vi "E727_Simple_Test.vi"(0 "System no.":i32=1 min=1 step=1, 2 "Interface":u16(ring) items=["RS232", "TCP/IP", "USB"], 3 "Timeout":u32=5000, 5 "error in":errorcluster, 6 "RS232 settings":cluster{"Portnumber":i32, "Baudrate":u16}={"Portnumber"=0, "Baudrate"=5} {"Baudrate" items=["9600", "14400", "19200", "38400", "57600", "115200"]; "Portnumber" items=["COM1", "COM2", "COM3", "COM4", "COM5", "COM6", "COM7", "COM8", "COM9", "COM10", "COM11", "COM12", "COM13", "COM14", "COM15", "COM16", "COM17", "COM18", "COM19", "COM20", "COM21", "COM22", "COM23", "COM24", "COM25", "COM26", "COM27", "COM28", "COM29", "COM30"]}, 7 "TCP/IP settings":T1={"Host address/name"="localhost", "Port"=50000, "Board"=0, "TCP/IP Search?"=TRUE}, 8 "USB settings":cluster{"S/N":string, "USB Search?":bool}={"S/N"="", "USB Search?"=TRUE}) -> (14 "Identification":string, 15 "Helpstring":string, 16 "Conn. Axes":string[](array[string]), 17 "Position":dbl[](array[numeric]) format="%.6f", 19 "error out":errorcluster)   [LabVIEW 2014]
doc: "This simple test VI is a stand-alone sample application. Use the \nHelp->Show Context Help menu sequence in the LabVIEW environment to display the Context Help window with the VI and control/indicator descriptions.\nSpecify \n- System no. (= 1 in a one-system configuration),\n- Interface (= RS232, TCP/IP or USB)\n- Timeout value (in milliseconds)\n- and interface settings first.\nThen start the VI. The VI will open a connection to the E-727 and query the controller for its identification string (*IDN?), help string (HLP?), the IDs (SAI?) and stage names (CST?) of the connected axes and their current position values (POS?). The diagram shows how to combine the driver and support VIs for these tasks."
panel:
  out "Stage names":string[](array[string])
  # "Simple E-727 communication test program"
  # "Select E-727 interface, timeout value and interface settings first, then start the VI. \nThe VI will open the chosen port, query for the connected axes (SAI?), the stage names (CST?), the position (POS?), Identification (*IDN?) and help string\n(HLP?). See VI and control/ indicator information for details."
  # "Only for\nInterface = \nTCP/IP:"
  # "Only for\nInterface = \nRS232:"
  # "Only for\nInterface = \nUSB:"
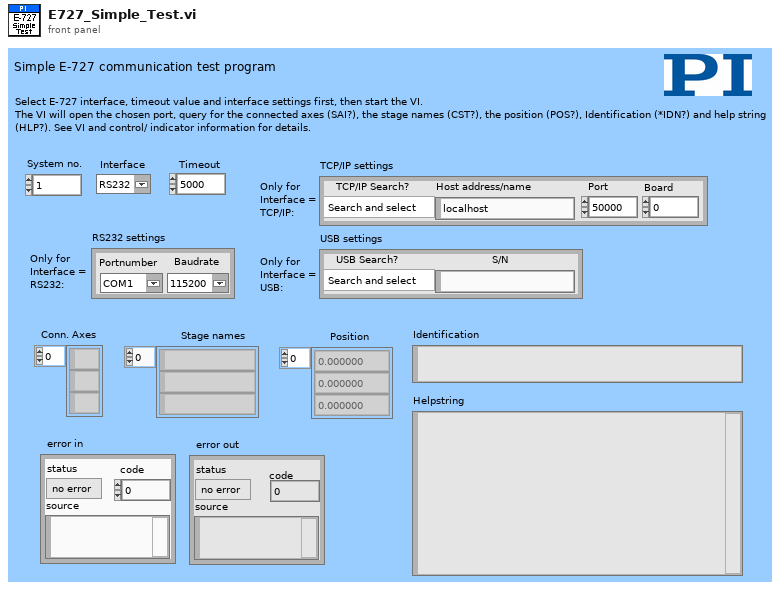
[diagram p1: front panel]
types:
  T1 = cluster{"Host address/name":string, "Port":i32, "Board":i32, "TCP/IP Search?":bool}
  T2 = cluster{"Host address/name":string, "Port":i32, "Board":i32}
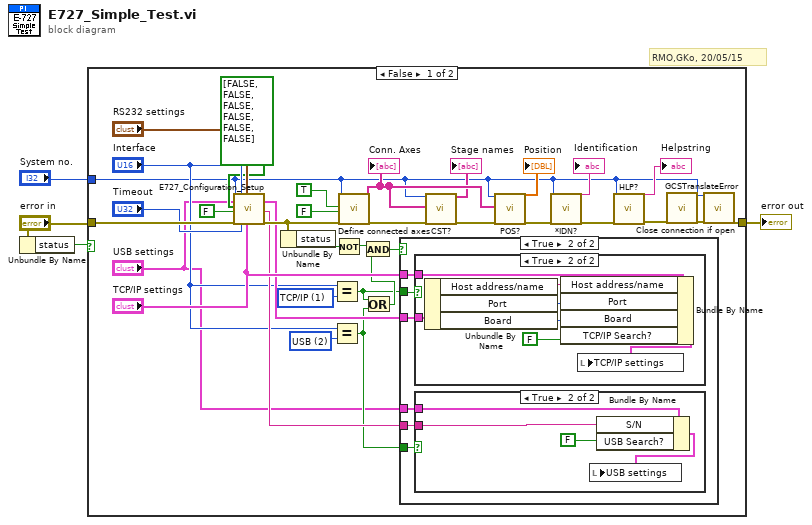
[diagram p0: block diagram]
diagram:
  # "RMO,GKo, 20/05/15"
  n1 = Unbundle By Name("error in") -> ("status"=w2:bool)
  n2 = case shown="False" w2 {
    tunnel: [w6 w56] -> w3
    tunnel: "error in" -> [w26 w56]
    tunnel: "System no." -> [w5 _]
    frame False {
      w13 = u16 2 items=["RS232", "TCP/IP", "USB"] ("Interface")
      w14 = u16 1 items=["RS232", "TCP/IP", "USB"] ("Interface")
      n3 = call "E727_Configuration_Setup.vi"("System no."=w5, "USB settings"="USB settings", "Are stages connected?"=bool[] [FALSE, FALSE, FALSE, FALSE, FALSE, FALSE], "Change servo status to ON?"=FALSE ("Connected?"), "error in"=w26, "Interface"="Interface", "Timeout"="Timeout", "RS232 settings"="RS232 settings", "TCP/IP settings"="TCP/IP settings") -> ("TCP/IP settings out"=w17:T2, "USB: S/N out"=w16:string, "error out"=w22:errorcluster)  [unwired: 5 in, 3 out]
      n4 = Unbundle By Name(w22) -> ("status"=w21:bool)
      n5 = Equal?(x="Interface", y=w14) -> (x = y?=w11:bool)
      n6 = Equal?(x="Interface", y=w13) -> (x = y?=w10:bool)
      n7 = Not(x=w21) -> (.not. x?=w19:bool)
      n8 = call "Define connected axes.vi"("System no."=w5, "Read from\ncontroller?"=TRUE ("Read from\nController"), "Invert\norder?"=FALSE ("Invert\nOrder"), "error in"=w22) -> ("Conn. Axes out"=w28:string[], "error out"=w30:errorcluster)  [unwired: 1 in, 13 out]
      "Conn. Axes" <- w28
      n9 = Or(x=w11, y=w10) -> (x .or. y?=w12:bool)
      n10 = And(x=w19, y=w12) -> (x .and. y?=w20:bool)
      n11 = case shown="True" w20 {
        tunnel: "TCP/IP settings" -> [_ w44]
        tunnel: w17 -> [_ w43]
        tunnel: w16 -> [_ w41]
        tunnel: "USB settings" -> [_ w42]
        tunnel: w11 -> [_ w40]
        tunnel: w10 -> [_ w39]
        frame False {
        }
        frame True {
          n12 = case shown="True" w40 {
            tunnel: w44 -> [_ w54]
            tunnel: w43 -> [_ w52]
            frame False {
            }
            frame True {
              n13 = Unbundle By Name(w52) -> ("Host address/name"=w51:string, "Port"=w50:i32, "Board"=w49:i32)
              n14 = Bundle By Name(cluster=w54, "Host address/name"=w51, "Port"=w50, "Board"=w49, "TCP/IP Search?"=FALSE) -> (w55:T1)
              n15 = local write "TCP/IP settings"(w55) -> ()
            }
          }
          n16 = case shown="True" w39 {
            tunnel: w42 -> [_ w48]
            tunnel: w41 -> [_ w46]
            frame False {
            }
            frame True {
              n17 = Bundle By Name(cluster=w48, "S/N"=w46, "USB Search?"=FALSE ("TCP/IP Search?")) -> (w45:cluster{"S/N":string, "USB Search?":bool})
              n18 = local write "USB settings"(w45) -> ()
            }
          }
        }
      }
      n19 = call "CST?.vi"("System no."=w5, "Axes to query"=w28, "error in"=w30) -> ("Stage names"=→"Stage names":string[], "error out"=w29:errorcluster)  [unwired: 2 in, 13 out]
      n20 = call "POS?.vi"("System no."=w5, "Axes to query"=w28, "error in"=w29) -> ("Position"=→"Position":dbl[], "error out"=w32:errorcluster)  [unwired: 2 in, 13 out]
      n21 = call "*IDN?.vi"("System no."=w5, "error in"=w32) -> ("Identification"=→"Identification":string, "error out"=w38:errorcluster)  [unwired: 16 out]
      n22 = call "HLP?.vi"("System no."=w5, "error in"=w38) -> ("Help string"=→"Helpstring":string, "error out"=w31:errorcluster)  [unwired: 16 out]
      n23 = call "GCSTranslateError.vi"("error in"=w31) -> ("error out"=w7:errorcluster)  [unwired: 18 out]
      n24 = call "Close connection if open.vi"("System no."=w5, "error in"=w7) -> ("error out"=w6:errorcluster)  [unwired: 1 in, 16 out]
    }
    frame True {
    }
  }
  "error out" <- w3
